vi "ALTS-2015 Test Type Pulse Count Calc.vi"(10 "Desired Test Type":i32, 11 "Current Test Type":i32) -> (3 "No. of Pulses Required":i32)   [LabVIEW 2013]
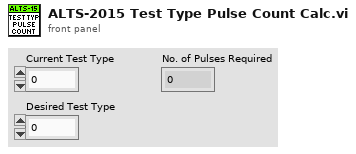
[diagram p1: front panel]
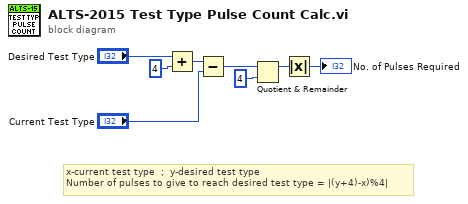
[diagram p0: block diagram]
diagram:
  # "x-current test type  ;  y-desired test type\nNumber of pulses to give to reach desired test type = |(y+4)-x)%4|"
  n1 = Add(x="Desired Test Type", y=4) -> (x+y=w2:i32)
  n2 = Subtract(x=w2, y="Current Test Type") -> (x-y=w3:i32)
  n3 = Quotient & Remainder(x=w3, y=4) -> (x-y*floor(x/y)=w5:i32)  [unwired: 1 out]
  n4 = Absolute Value(x=w5) -> (abs(x)=→"No. of Pulses Required":i32)
